vi "Build SWD.vi"(9 "status word flags":T1, 10 "RT Address":u16) -> (3 "swd":u8[](array[numeric]) format="%.0x")   [LabVIEW 2020, in "Ballard_1553_Hardware_ni.lvlib"]
uses:
  Ballard_1553_Hardware_ni.lvlib
  _typedefs/sw_flags.ctl
panel:
  out "swd u16":u16 format="%.0x"
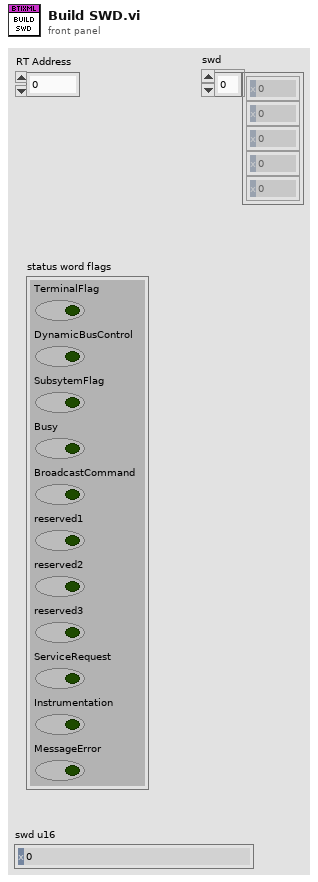
[diagram p1: front panel]
types:
  T1 = typedef "Ballard_1553_Hardware_ni.lvlib/sw_flags.ctl" = cluster{"TerminalFlag":bool, "DynamicBusControl":bool, "SubsytemFlag":bool, "Busy":bool, "BroadcastCommand":bool, "reserved1":bool, "reserved2":bool, "reserved3":bool, "ServiceRequest":bool, "Instrumentation":bool, "MessageError":bool}
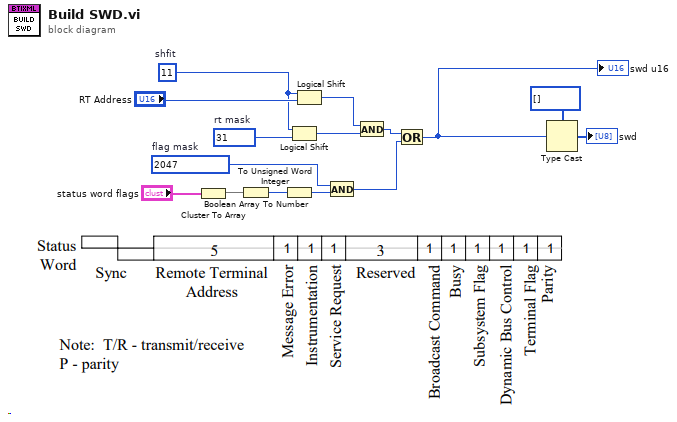
[diagram p0: block diagram]
diagram:
  w9 = i16 11  # shfit
  w15 = u16 31  # rt mask
  w7 = u16 2047  # flag mask
  n1 = Cluster To Array(cluster="status word flags") -> (array=w10:bool[])
  n2 = Boolean Array To Number(Boolean array=w10) -> (number=w8:u32)
  n3 = To Unsigned Word Integer(number=w8) -> (unsigned 16bit integer=w4:u16)
  n4 = Logical Shift(y=w9, x=w15) -> (x << y=w13:u16)
  n5 = Logical Shift(y=w9, x="RT Address") -> (x << y=w14:u16)
  n6 = And(x=w7, y=w4) -> (x .and. y?=w5:u16)
  n7 = And(x=w14, y=w13) -> (x .and. y?=w6:u16)
  n8 = Or(x=w6, y=w5) -> (x .or. y?=w3:u16)
  "swd u16" <- w3
  n9 = Type Cast(type=u8[] [], x=w3) -> (*(type *) &x=→"swd":u8[])
